vi "Read Single Digital Input.vi"(0 "Line":tag, 5 "Expected Data":bool, 11 "Error In":errorcluster) -> (4 "Pass/Fail?":bool, 6 "Report Text":string, 8 "Data":bool, 15 "Error Out":errorcluster)   [LabVIEW 2016]
uses:
  <vilib>/DAQmx/read.llb/DAQmx Read (Digital Bool 1Line 1Point).vi
  <vilib>/DAQmx/create/channels.llb/DAQmx Create Channel (DI-Digital Input).vi
  <vilib>/DAQmx/miscellaneous.llb/DAQmx Fill In Error Info.vi
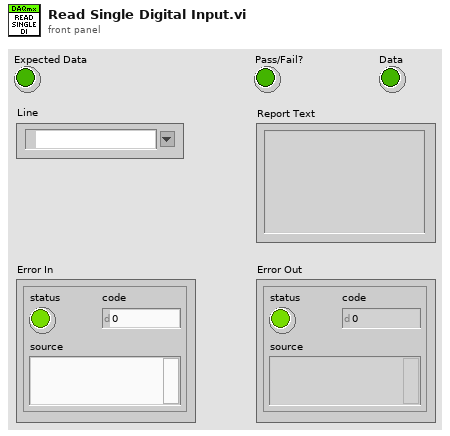
[diagram p1: front panel]
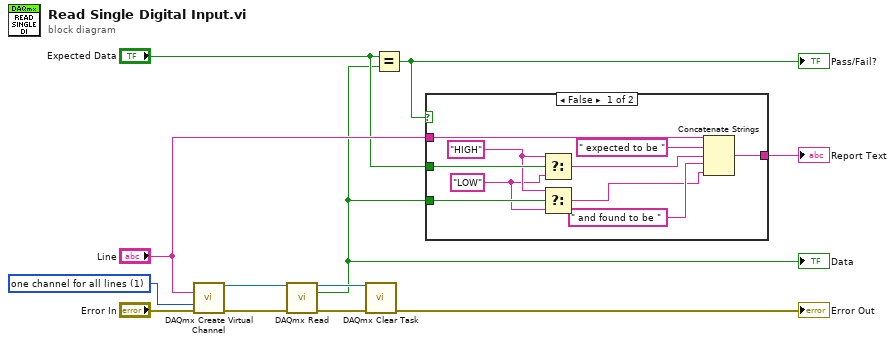
[diagram p0: block diagram]
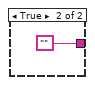
[diagram p2: hidden frame]
diagram:
  w12 = 1 items=["one channel for each line", "one channel for all lines"] ("line grouping")
  n1 = call-poly <vilib>:"DAQmx Create Virtual Channel.vi"("lines"="Line", "line grouping"=w12, "error in"="Error In") -> ("task out"=w8:refnum<k21>, "error out"=w11:errorcluster)  [unwired: 11 in]
  n2 = call-poly <vilib>:"DAQmx Read.vi"("task/channels in"=w8, "error in"=w11) -> ("task out"=w9:refnum<k21>, "data"=w2:bool, "error out"=w10:errorcluster)  [unwired: 11 in]
  "Data" <- w2
  n3 = call <vilib>:"DAQmx Clear Task.vi"("task in"=w9, "error in"=w10) -> ("error out"=→"Error Out":errorcluster)  [unwired: 13 in]
  n4 = Equal?(x="Expected Data", y=w2) -> (x = y?=w5:bool)
  "Pass/Fail?" <- w5
  n5 = case shown="False" w5 {
    tunnel: "Line" -> [w20 _]
    tunnel: "Expected Data" -> [w22 _]
    tunnel: w2 -> [w21 _]
    tunnel: [w15 ""] -> w1
    frame False {
      w13 = "LOW" ("Report Text")
      w14 = "HIGH" ("Report Text")
      n6 = Select(t=w14, s=w22, f=w13) -> (s? t:f=w18:string)
      n7 = Select(t=w14, s=w21, f=w13) -> (s? t:f=w16:string)
      n8 = Concatenate Strings(w20, " expected to be " ("string"), w18, " and found to be " ("string"), w16) -> (w15:string)
    }
    frame True {
    }
  }
  "Report Text" <- w1
